vi "Nested Alias Unique.vi"(10 "Nested Alias":string, 11 "Self Actor":refnum<class "Self Actor.lvclass">) -> (0 "error out":errorcluster, 2 "Nested Alias Unique?":bool)   [LabVIEW 2021, in "jettl.lvlib" / "Self Actor.lvclass"]
uses:
  Self Actor.lvclass
  Self Actor.lvclass/Self Actor.ctl
  jettl.lvlib
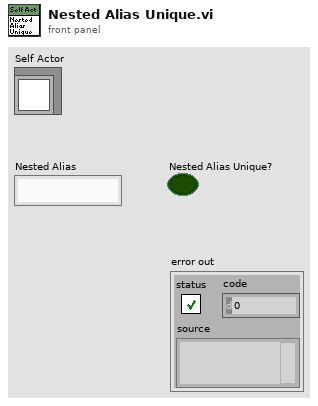
[diagram p1: front panel]
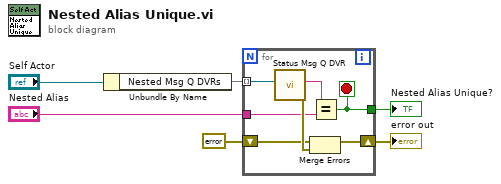
[diagram p0: block diagram]
diagram:
  n1 = Unbundle By Name("Self Actor") -> ("Nested Msg Q DVRs"=w2:set{refnum<data-value>})
  n2 = for {
    tunnel: w2 -> [w13] mode=indexing
    shift-right: [w11] -> w6
    shift-left: errorcluster {"status"=FALSE, "code"=0, "source"=""} ("error IO") -> [w10]
    tunnel: "Nested Alias" -> [w8]
    tunnel: [w7] -> w4
    stop <- w7 stop-if-true
    n3 = call "Status Msg Q DVR.vi"("Msg Q DVR"=w13) -> ("error out"=w12:errorcluster, "Msg Q DVR Alias"=w9:string)  [unwired: 9 in]
    n4 = Merge Errors(w10, w12) -> (w11:errorcluster)
    n5 = Equal?(x=w9, y=w8) -> (x = y?=w7:bool)
  }
  "error out" <- w6
  "Nested Alias Unique?" <- w4
